vi "Global 1.vi"() -> ()   [LabVIEW 2017]
panel:
  in  "Global Value":dbl
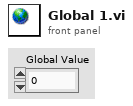
[diagram p1: front panel]
diagram:
